vi "ReleaseQueues.vi"(9 "Force destroy (F)":bool, 11 "queue cluster":T1) -> (0 "error out":errorcluster)   [LabVIEW 2014]
uses:
  typedefs/QueueCluster.ctl
  typedefs/clientStatus.ctl
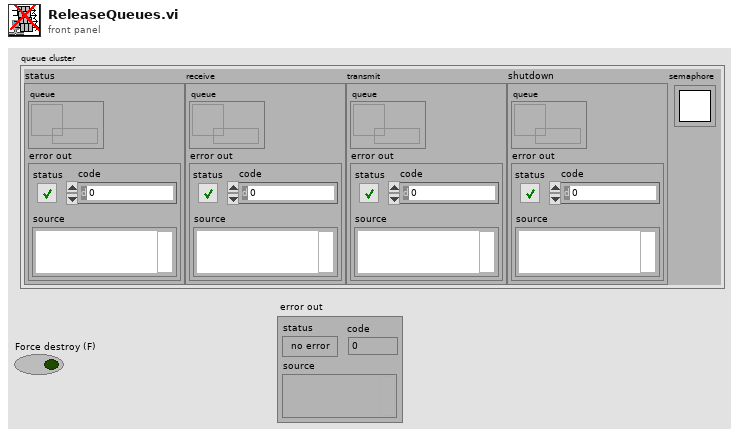
[diagram p1: front panel]
types:
  T1 = typedef "QueueCluster.ctl" = cluster{"status":cluster{"queue":refnum<queue>, "error out":errorcluster}, "receive":cluster{"queue":refnum<queue>, "error out":errorcluster}, "transmit":cluster{"queue":refnum<queue>, "error out":errorcluster}, "shutdown":cluster{"queue":refnum<queue>, "error out":errorcluster}, "semaphore":T2}
  T2 = typedef "Semaphore RefNum" = refnum<k1>
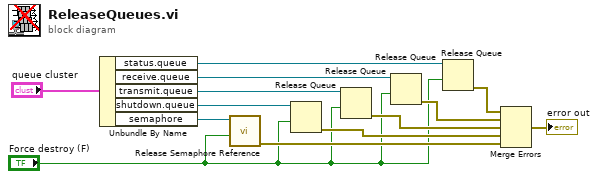
[diagram p0: block diagram]
diagram:
  n1 = Unbundle By Name("queue cluster") -> ("status.queue"=w11:refnum<queue>, "receive.queue"=w8:refnum<queue>, "transmit.queue"=w7:refnum<queue>, "shutdown.queue"=w3:refnum<queue>, "semaphore"=w9:T2)
  n2 = call <vilib>:"Release Semaphore Reference.vi"("force destroy? (F)"="Force destroy (F)", "semaphore"=w9) -> ("error out"=w4:errorcluster)  [unwired: 8 in, 1 out]
  n3 = Release Queue(queue=w3, force destroy? (F)="Force destroy (F)") -> (error out=w2:errorcluster)  [unwired: 1 in, 2 out]
  n4 = Release Queue(queue=w7, force destroy? (F)="Force destroy (F)") -> (error out=w5:errorcluster)  [unwired: 1 in, 2 out]
  n5 = Release Queue(queue=w8, force destroy? (F)="Force destroy (F)") -> (error out=w6:errorcluster)  [unwired: 1 in, 2 out]
  n6 = Release Queue(queue=w11, force destroy? (F)="Force destroy (F)") -> (error out=w10:errorcluster)  [unwired: 1 in, 2 out]
  n7 = Merge Errors(w10, w6, w5, w2, w4) -> (→"error out":errorcluster)
